vi "ReadForceIni2#.vi"(1 "configuration file path":path=path "E:/LabVIEW/福尔达/AppData") -> ()   [LabVIEW 2018]
uses:
  <vilib>/Utility/config.llb/Read Key (String).vi
  <vilib>/Utility/config.llb/Read Key (Double).vi
  <vilib>/Utility/config.llb/NI_LVConfig.lvlib
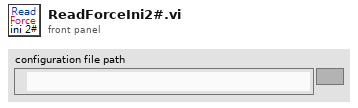
[diagram p1: front panel]
types:
  T1 = typedef "NI_LVConfig.lvlib/Config Data RefNum.ctl" = refnum<k1>
  T2 = cluster{"选择":enum16{"Fx", "Fy", "Fz", "Mx", "My", "Mz"}, "系数x":sgl, "系数+":sgl, "上限":sgl, "下限":sgl, "Ymax":dbl, "Ymin":dbl, "点数":dbl, "锁系数x":sgl, "锁上限":sgl, "锁下限":sgl, "锁系数+":sgl, "起点":dbl, "终点":dbl, "锁起点":dbl, "锁终点":dbl, "上参考":sgl, "下参考":sgl, "基准":sgl}
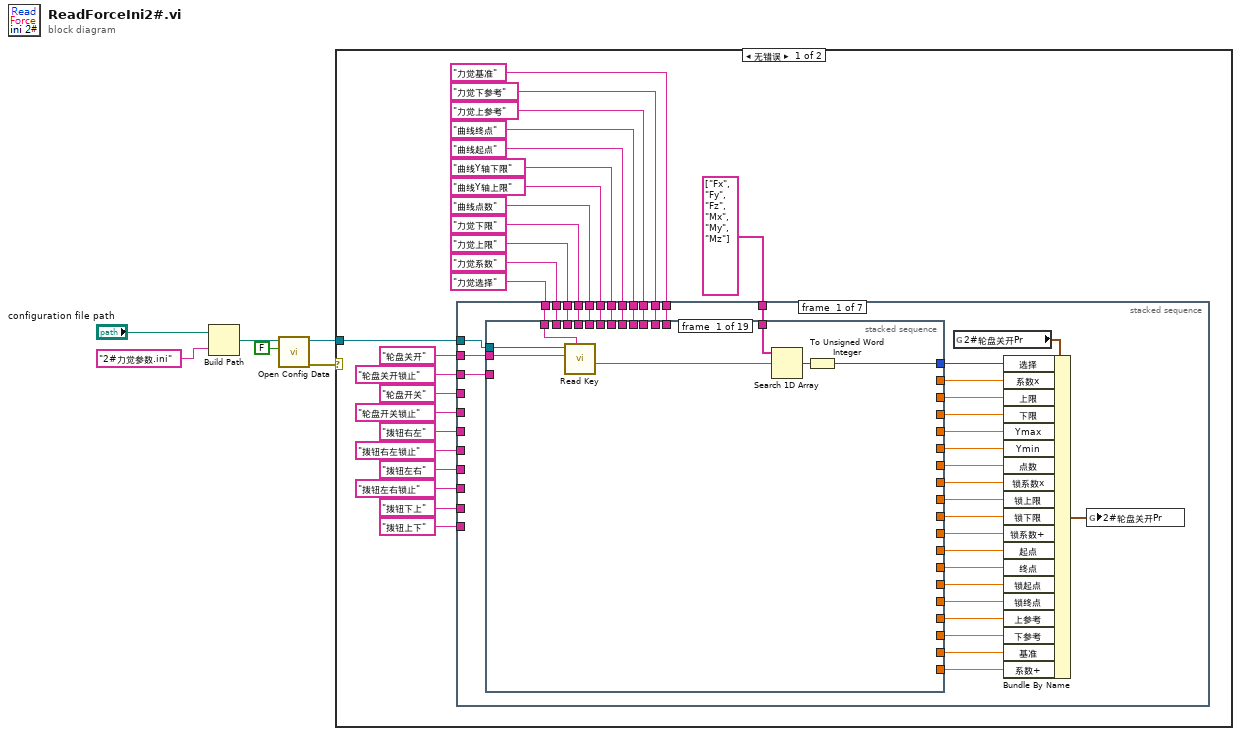
[diagram p0: block diagram]
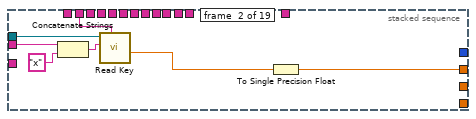
[diagram p2: hidden frame]
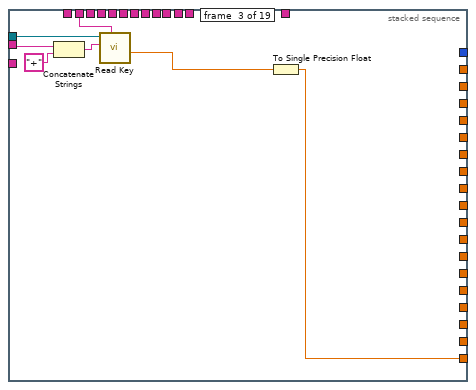
[diagram p3: hidden frame]
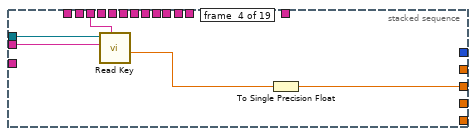
[diagram p4: hidden frame]
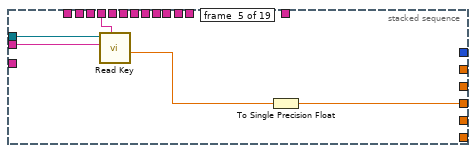
[diagram p5: hidden frame]
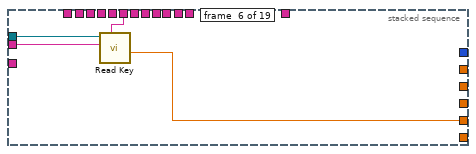
[diagram p6: hidden frame]
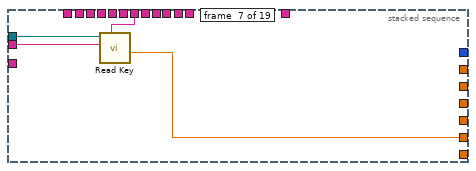
[diagram p7: hidden frame]
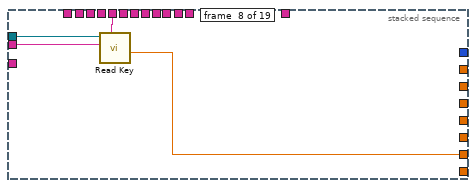
[diagram p8: hidden frame]
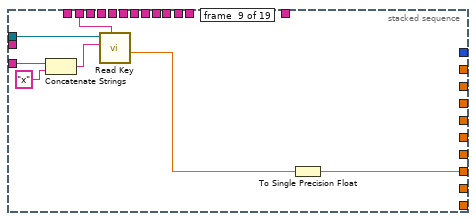
[diagram p9: hidden frame]
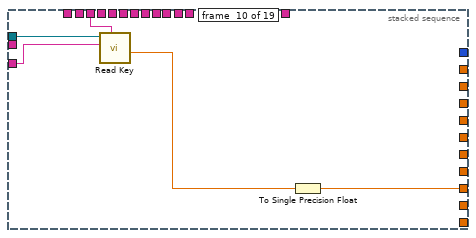
[diagram p10: hidden frame]
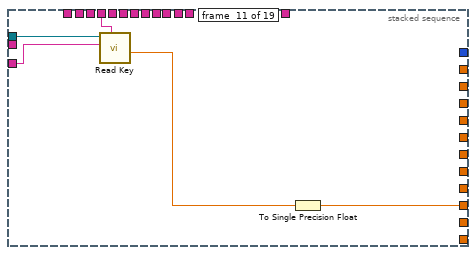
[diagram p11: hidden frame]
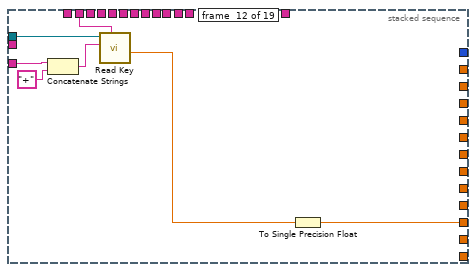
[diagram p12: hidden frame]
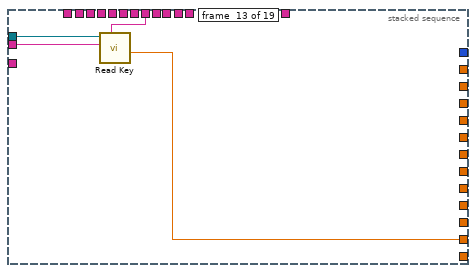
[diagram p13: hidden frame]
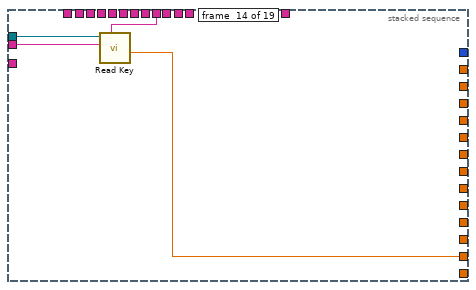
[diagram p14: hidden frame]
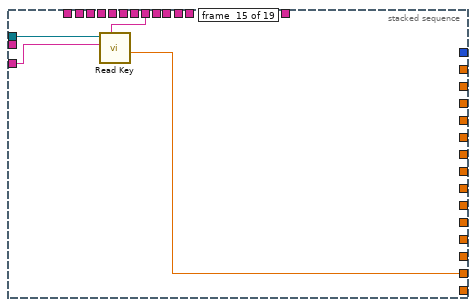
[diagram p15: hidden frame]
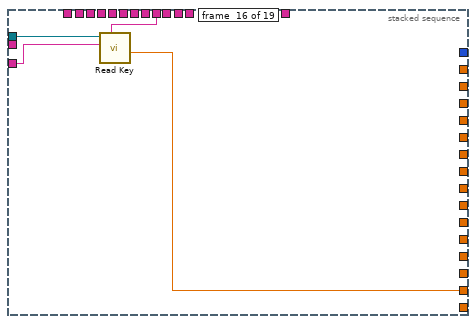
[diagram p16: hidden frame]
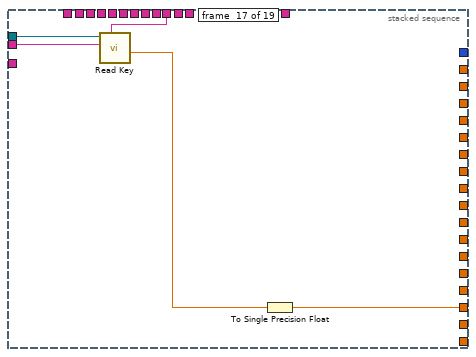
[diagram p17: hidden frame]
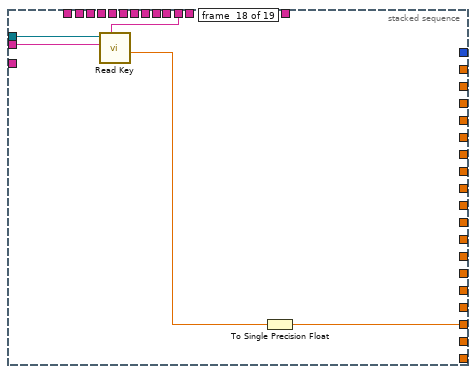
[diagram p18: hidden frame]
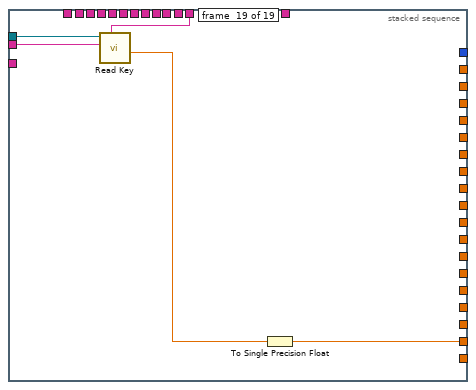
[diagram p19: hidden frame]
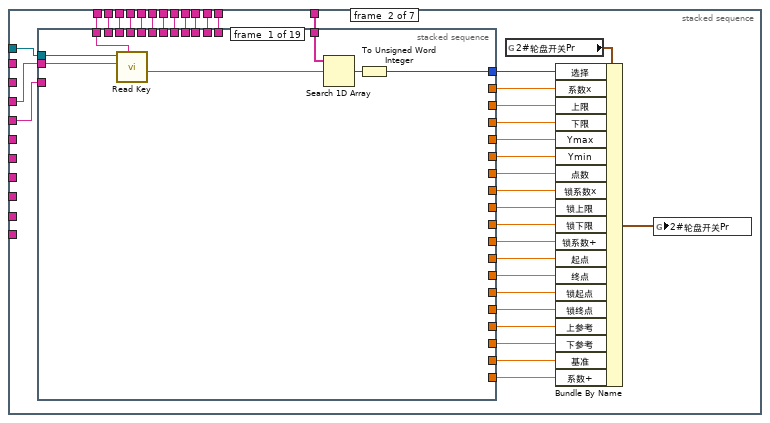
[diagram p20: hidden frame]
diagram:
  n1 = Build Path(base path="configuration file path", name or relative path="2#力觉参数.ini" ("名称或相对路径")) -> (appended path=w3:path)
  n2 = call <vilib>:"Open Config Data.vi"("create file if necessary (T)"=FALSE, "configuration file path"=w3) -> ("error out"=w1:errorcluster, "refnum"=w5:T1)  [unwired: 7 in, 1 out]
  n3 = case shown="无错误" w1 {
    tunnel: w5 -> [w12 w765]
    frame No Error {
      n4 = stacked-sequence {
        tunnel: string[] ["Fx", "Fy", "Fz", "Mx", "My", "Mz"] -> [w67 w202 w337 w472 w600 w696 _]
        tunnel: "轮盘关开" -> [w62 _ _ _ _ _ _]
        tunnel: w12 -> [w66 w201 w336 w471 w599 w695 w763]
        tunnel: "力觉选择" -> [w61 w197 w332 w467 w595 w691 _]
        tunnel: "力觉系数" -> [w60 w196 w331 w466 w594 w690 _]
        tunnel: "力觉上限" -> [w59 w195 w330 w465 w593 w689 _]
        tunnel: "力觉下限" -> [w58 w194 w329 w464 w592 w688 _]
        tunnel: "曲线点数" -> [w57 w193 w328 w463 w591 w687 _]
        tunnel: "曲线Y轴上限" -> [w56 w192 w327 w462 w590 w686 _]
        tunnel: "曲线Y轴下限" -> [w55 w191 w326 w461 w589 w685 _]
        tunnel: "拨钮下上" -> [_ _ _ _ w571 _ _]
        tunnel: "拨钮上下" -> [_ _ _ _ _ w667 _]
        tunnel: "曲线起点" -> [w54 w190 w325 w460 w588 w684 _]
        tunnel: "曲线终点" -> [w53 w189 w324 w459 w587 w683 _]
        tunnel: "力觉上参考" -> [w38 w174 w309 w444 w578 w674 _]
        tunnel: "力觉下参考" -> [w37 w173 w308 w443 w575 w671 _]
        tunnel: "力觉基准" -> [w33 w169 w304 w439 w573 w669 _]
        tunnel: "轮盘关开锁止" -> [w31 _ _ _ _ _ _]
        tunnel: "轮盘开关" -> [_ w167 _ _ _ _ _]
        tunnel: "轮盘开关锁止" -> [_ w166 _ _ _ _ _]
        tunnel: "拨钮右左" -> [_ _ w302 _ _ _ _]
        tunnel: "拨钮左右" -> [_ _ _ w437 _ _ _]
        tunnel: "拨钮左右锁止" -> [_ _ _ w436 _ _ _]
        tunnel: "拨钮右左锁止" -> [_ _ w301 _ _ _ _]
        frame #0 {
          n5 = stacked-sequence {
            tunnel: w67 -> [w74 _ _ _ _ _ _ _ _ _ _ _ _ _ _ _ _ _ _]
            tunnel: w62 -> [w72 w76 w83 w93 w98 w102 w106 w110 _ _ _ _ w135 w139 _ _ w154 w159 w164]
            tunnel: w66 -> [w71 w81 w88 w92 w97 w101 w105 w109 w117 w122 w127 w134 w138 w142 w146 w150 w155 w160 w165]
            tunnel: [w70 _ _ _ _ _ _ _ _ _ _ _ _ _ _ _ _ _ _] -> w64
            tunnel: w61 -> [w68 _ _ _ _ _ _ _ _ _ _ _ _ _ _ _ _ _ _]
            tunnel: w60 -> [_ w80 w87 _ _ _ _ _ w116 _ _ w129 _ _ _ _ _ _ _]
            tunnel: w59 -> [_ _ _ w89 _ _ _ _ _ w119 _ _ _ _ _ _ _ _ _]
            tunnel: w58 -> [_ _ _ _ w94 _ _ _ _ _ w124 _ _ _ _ _ _ _ _]
            tunnel: w57 -> [_ _ _ _ _ _ _ w108 _ _ _ _ _ _ _ _ _ _ _]
            tunnel: w56 -> [_ _ _ _ _ w100 _ _ _ _ _ _ _ _ _ _ _ _ _]
            tunnel: w55 -> [_ _ _ _ _ _ w103 _ _ _ _ _ _ _ _ _ _ _ _]
            tunnel: w54 -> [_ _ _ _ _ _ _ _ _ _ _ _ w137 _ w144 _ _ _ _]
            tunnel: w53 -> [_ _ _ _ _ _ _ _ _ _ _ _ _ w140 _ w149 _ _ _]
            tunnel: [_ w78 _ _ _ _ _ _ _ _ _ _ _ _ _ _ _ _ _] -> w52
            tunnel: [_ _ _ w90 _ _ _ _ _ _ _ _ _ _ _ _ _ _ _] -> w51
            tunnel: [_ _ _ _ w95 _ _ _ _ _ _ _ _ _ _ _ _ _ _] -> w50
            tunnel: [_ _ _ _ _ w99 _ _ _ _ _ _ _ _ _ _ _ _ _] -> w49
            tunnel: [_ _ _ _ _ _ w104 _ _ _ _ _ _ _ _ _ _ _ _] -> w48
            tunnel: [_ _ _ _ _ _ _ w107 _ _ _ _ _ _ _ _ _ _ _] -> w47
            tunnel: [_ _ _ _ _ _ _ _ w113 _ _ _ _ _ _ _ _ _ _] -> w46
            tunnel: [_ _ _ _ _ _ _ _ _ w120 _ _ _ _ _ _ _ _ _] -> w45
            tunnel: [_ _ _ _ _ _ _ _ _ _ w125 _ _ _ _ _ _ _ _] -> w44
            tunnel: [_ _ _ _ _ _ _ _ _ _ _ w132 _ _ _ _ _ _ _] -> w43
            tunnel: [_ _ _ _ _ _ _ _ _ _ _ _ w136 _ _ _ _ _ _] -> w42
            tunnel: [_ _ _ _ _ _ _ _ _ _ _ _ _ w141 _ _ _ _ _] -> w41
            tunnel: [_ _ _ _ _ _ _ _ _ _ _ _ _ _ w145 _ _ _ _] -> w40
            tunnel: [_ _ _ _ _ _ _ _ _ _ _ _ _ _ _ w148 _ _ _] -> w39
            tunnel: w38 -> [_ _ _ _ _ _ _ _ _ _ _ _ _ _ _ _ w151 _ _]
            tunnel: w37 -> [_ _ _ _ _ _ _ _ _ _ _ _ _ _ _ _ _ w157 _]
            tunnel: [_ _ _ _ _ _ _ _ _ _ _ _ _ _ _ _ w153 _ _] -> w36
            tunnel: [_ _ _ _ _ _ _ _ _ _ _ _ _ _ _ _ _ w156 _] -> w35
            tunnel: [_ _ _ _ _ _ _ _ _ _ _ _ _ _ _ _ _ _ w162] -> w34
            tunnel: w33 -> [_ _ _ _ _ _ _ _ _ _ _ _ _ _ _ _ _ _ w161]
            tunnel: [_ _ w85 _ _ _ _ _ _ _ _ _ _ _ _ _ _ _ _] -> w32
            tunnel: w31 -> [_ _ _ _ _ _ _ _ w111 w118 w123 w128 _ _ w143 w147 _ _ _]
            frame #0 {
              n6 = call-poly <vilib>:"Read Key.vi"("section"=w68, "key"=w72, "refnum"=w71) -> ("value"=w73:string)  [unwired: 5 in, 3 out]
              n7 = Search 1D Array(1D array=w74, element=w73) -> (index of element=w69:i32)  [unwired: 1 in]
              n8 = To Unsigned Word Integer(number=w69) -> (unsigned 16bit integer=w70:u16)
            }
            frame #1 {
              n9 = Concatenate Strings(w76, "x") -> (w75:string)
              n10 = call-poly <vilib>:"Read Key.vi"("section"=w80, "key"=w75, "refnum"=w81) -> ("value"=w79:dbl)  [unwired: 5 in, 3 out]
              n11 = To Single Precision Float(number=w79) -> (single precision float=w78:sgl)
            }
            frame #2 {
              n12 = Concatenate Strings(w83, "+") -> (w82:string)
              n13 = call-poly <vilib>:"Read Key.vi"("section"=w87, "key"=w82, "refnum"=w88) -> ("value"=w86:dbl)  [unwired: 5 in, 3 out]
              n14 = To Single Precision Float(number=w86) -> (single precision float=w85:sgl)
            }
            frame #3 {
              n15 = call-poly <vilib>:"Read Key.vi"("section"=w89, "key"=w93, "refnum"=w92) -> ("value"=w91:dbl)  [unwired: 5 in, 3 out]
              n16 = To Single Precision Float(number=w91) -> (single precision float=w90:sgl)
            }
            frame #4 {
              n17 = call-poly <vilib>:"Read Key.vi"("section"=w94, "key"=w98, "refnum"=w97) -> ("value"=w96:dbl)  [unwired: 5 in, 3 out]
              n18 = To Single Precision Float(number=w96) -> (single precision float=w95:sgl)
            }
            frame #5 {
              n19 = call-poly <vilib>:"Read Key.vi"("section"=w100, "key"=w102, "refnum"=w101) -> ("value"=w99:dbl)  [unwired: 5 in, 3 out]
            }
            frame #6 {
              n20 = call-poly <vilib>:"Read Key.vi"("section"=w103, "key"=w106, "refnum"=w105) -> ("value"=w104:dbl)  [unwired: 5 in, 3 out]
            }
            frame #7 {
              n21 = call-poly <vilib>:"Read Key.vi"("section"=w108, "key"=w110, "refnum"=w109) -> ("value"=w107:dbl)  [unwired: 5 in, 3 out]
            }
            frame #8 {
              n22 = Concatenate Strings(w111, "x") -> (w115:string)
              n23 = call-poly <vilib>:"Read Key.vi"("section"=w116, "key"=w115, "refnum"=w117) -> ("value"=w112:dbl)  [unwired: 5 in, 3 out]
              n24 = To Single Precision Float(number=w112) -> (single precision float=w113:sgl)
            }
            frame #9 {
              n25 = call-poly <vilib>:"Read Key.vi"("section"=w119, "key"=w118, "refnum"=w122) -> ("value"=w121:dbl)  [unwired: 5 in, 3 out]
              n26 = To Single Precision Float(number=w121) -> (single precision float=w120:sgl)
            }
            frame #10 {
              n27 = call-poly <vilib>:"Read Key.vi"("section"=w124, "key"=w123, "refnum"=w127) -> ("value"=w126:dbl)  [unwired: 5 in, 3 out]
              n28 = To Single Precision Float(number=w126) -> (single precision float=w125:sgl)
            }
            frame #11 {
              n29 = Concatenate Strings(w128, "+") -> (w131:string)
              n30 = call-poly <vilib>:"Read Key.vi"("section"=w129, "key"=w131, "refnum"=w134) -> ("value"=w133:dbl)  [unwired: 5 in, 3 out]
              n31 = To Single Precision Float(number=w133) -> (single precision float=w132:sgl)
            }
            frame #12 {
              n32 = call-poly <vilib>:"Read Key.vi"("section"=w137, "key"=w135, "refnum"=w138) -> ("value"=w136:dbl)  [unwired: 5 in, 3 out]
            }
            frame #13 {
              n33 = call-poly <vilib>:"Read Key.vi"("section"=w140, "key"=w139, "refnum"=w142) -> ("value"=w141:dbl)  [unwired: 5 in, 3 out]
            }
            frame #14 {
              n34 = call-poly <vilib>:"Read Key.vi"("section"=w144, "key"=w143, "refnum"=w146) -> ("value"=w145:dbl)  [unwired: 5 in, 3 out]
            }
            frame #15 {
              n35 = call-poly <vilib>:"Read Key.vi"("section"=w149, "key"=w147, "refnum"=w150) -> ("value"=w148:dbl)  [unwired: 5 in, 3 out]
            }
            frame #16 {
              n36 = call-poly <vilib>:"Read Key.vi"("section"=w151, "key"=w154, "refnum"=w155) -> ("value"=w152:dbl)  [unwired: 5 in, 3 out]
              n37 = To Single Precision Float(number=w152) -> (single precision float=w153:sgl)
            }
            frame #17 {
              n38 = call-poly <vilib>:"Read Key.vi"("section"=w157, "key"=w159, "refnum"=w160) -> ("value"=w158:dbl)  [unwired: 5 in, 3 out]
              n39 = To Single Precision Float(number=w158) -> (single precision float=w156:sgl)
            }
            frame #18 {
              n40 = call-poly <vilib>:"Read Key.vi"("section"=w161, "key"=w164, "refnum"=w165) -> ("value"=w163:dbl)  [unwired: 5 in, 3 out]
              n41 = To Single Precision Float(number=w163) -> (single precision float=w162:sgl)
            }
          }
          n42 = global read "全局F参数.vi" "2#轮盘关开Pr"() -> (w65:T2)
          n43 = Bundle By Name(cluster=w65, "选择"=w64, "系数x"=w52, "上限"=w51, "下限"=w50, "Ymax"=w49, "Ymin"=w48, "点数"=w47, "锁系数x"=w46, "锁上限"=w45, "锁下限"=w44, "锁系数+"=w43, "起点"=w42, "终点"=w41, "锁起点"=w40, "锁终点"=w39, "上参考"=w36, "下参考"=w35, "基准"=w34, "系数+"=w32) -> (w63:T2)
          n44 = global write "全局F参数.vi" "2#轮盘关开Pr"(w63) -> ()
        }
        frame #1 {
          n45 = stacked-sequence {
            tunnel: w202 -> [w209 _ _ _ _ _ _ _ _ _ _ _ _ _ _ _ _ _ _]
            tunnel: w167 -> [w207 w211 w218 w228 w233 w237 w241 w245 _ _ _ _ w270 w274 _ _ w289 w294 w299]
            tunnel: w201 -> [w206 w216 w223 w227 w232 w236 w240 w244 w252 w257 w262 w269 w273 w277 w281 w285 w290 w295 w300]
            tunnel: [w205 _ _ _ _ _ _ _ _ _ _ _ _ _ _ _ _ _ _] -> w199
            tunnel: w197 -> [w203 _ _ _ _ _ _ _ _ _ _ _ _ _ _ _ _ _ _]
            tunnel: w196 -> [_ w215 w222 _ _ _ _ _ w251 _ _ w264 _ _ _ _ _ _ _]
            tunnel: w195 -> [_ _ _ w224 _ _ _ _ _ w254 _ _ _ _ _ _ _ _ _]
            tunnel: w194 -> [_ _ _ _ w229 _ _ _ _ _ w259 _ _ _ _ _ _ _ _]
            tunnel: w193 -> [_ _ _ _ _ _ _ w243 _ _ _ _ _ _ _ _ _ _ _]
            tunnel: w192 -> [_ _ _ _ _ w235 _ _ _ _ _ _ _ _ _ _ _ _ _]
            tunnel: w191 -> [_ _ _ _ _ _ w238 _ _ _ _ _ _ _ _ _ _ _ _]
            tunnel: w190 -> [_ _ _ _ _ _ _ _ _ _ _ _ w272 _ w279 _ _ _ _]
            tunnel: w189 -> [_ _ _ _ _ _ _ _ _ _ _ _ _ w275 _ w284 _ _ _]
            tunnel: [_ w213 _ _ _ _ _ _ _ _ _ _ _ _ _ _ _ _ _] -> w188
            tunnel: [_ _ _ w225 _ _ _ _ _ _ _ _ _ _ _ _ _ _ _] -> w187
            tunnel: [_ _ _ _ w230 _ _ _ _ _ _ _ _ _ _ _ _ _ _] -> w186
            tunnel: [_ _ _ _ _ w234 _ _ _ _ _ _ _ _ _ _ _ _ _] -> w185
            tunnel: [_ _ _ _ _ _ w239 _ _ _ _ _ _ _ _ _ _ _ _] -> w184
            tunnel: [_ _ _ _ _ _ _ w242 _ _ _ _ _ _ _ _ _ _ _] -> w183
            tunnel: [_ _ _ _ _ _ _ _ w248 _ _ _ _ _ _ _ _ _ _] -> w182
            tunnel: [_ _ _ _ _ _ _ _ _ w255 _ _ _ _ _ _ _ _ _] -> w181
            tunnel: [_ _ _ _ _ _ _ _ _ _ w260 _ _ _ _ _ _ _ _] -> w180
            tunnel: [_ _ _ _ _ _ _ _ _ _ _ w267 _ _ _ _ _ _ _] -> w179
            tunnel: [_ _ _ _ _ _ _ _ _ _ _ _ w271 _ _ _ _ _ _] -> w178
            tunnel: [_ _ _ _ _ _ _ _ _ _ _ _ _ w276 _ _ _ _ _] -> w177
            tunnel: [_ _ _ _ _ _ _ _ _ _ _ _ _ _ w280 _ _ _ _] -> w176
            tunnel: [_ _ _ _ _ _ _ _ _ _ _ _ _ _ _ w283 _ _ _] -> w175
            tunnel: w174 -> [_ _ _ _ _ _ _ _ _ _ _ _ _ _ _ _ w286 _ _]
            tunnel: w173 -> [_ _ _ _ _ _ _ _ _ _ _ _ _ _ _ _ _ w292 _]
            tunnel: [_ _ _ _ _ _ _ _ _ _ _ _ _ _ _ _ w288 _ _] -> w172
            tunnel: [_ _ _ _ _ _ _ _ _ _ _ _ _ _ _ _ _ w291 _] -> w171
            tunnel: [_ _ _ _ _ _ _ _ _ _ _ _ _ _ _ _ _ _ w297] -> w170
            tunnel: w169 -> [_ _ _ _ _ _ _ _ _ _ _ _ _ _ _ _ _ _ w296]
            tunnel: [_ _ w220 _ _ _ _ _ _ _ _ _ _ _ _ _ _ _ _] -> w168
            tunnel: w166 -> [_ _ _ _ _ _ _ _ w246 w253 w258 w263 _ _ w278 w282 _ _ _]
            frame #0 {
              n46 = call-poly <vilib>:"Read Key.vi"("section"=w203, "key"=w207, "refnum"=w206) -> ("value"=w208:string)  [unwired: 5 in, 3 out]
              n47 = Search 1D Array(1D array=w209, element=w208) -> (index of element=w204:i32)  [unwired: 1 in]
              n48 = To Unsigned Word Integer(number=w204) -> (unsigned 16bit integer=w205:u16)
            }
            frame #1 {
              n49 = Concatenate Strings(w211, "x") -> (w210:string)
              n50 = call-poly <vilib>:"Read Key.vi"("section"=w215, "key"=w210, "refnum"=w216) -> ("value"=w214:dbl)  [unwired: 5 in, 3 out]
              n51 = To Single Precision Float(number=w214) -> (single precision float=w213:sgl)
            }
            frame #2 {
              n52 = Concatenate Strings(w218, "+") -> (w217:string)
              n53 = call-poly <vilib>:"Read Key.vi"("section"=w222, "key"=w217, "refnum"=w223) -> ("value"=w221:dbl)  [unwired: 5 in, 3 out]
              n54 = To Single Precision Float(number=w221) -> (single precision float=w220:sgl)
            }
            frame #3 {
              n55 = call-poly <vilib>:"Read Key.vi"("section"=w224, "key"=w228, "refnum"=w227) -> ("value"=w226:dbl)  [unwired: 5 in, 3 out]
              n56 = To Single Precision Float(number=w226) -> (single precision float=w225:sgl)
            }
            frame #4 {
              n57 = call-poly <vilib>:"Read Key.vi"("section"=w229, "key"=w233, "refnum"=w232) -> ("value"=w231:dbl)  [unwired: 5 in, 3 out]
              n58 = To Single Precision Float(number=w231) -> (single precision float=w230:sgl)
            }
            frame #5 {
              n59 = call-poly <vilib>:"Read Key.vi"("section"=w235, "key"=w237, "refnum"=w236) -> ("value"=w234:dbl)  [unwired: 5 in, 3 out]
            }
            frame #6 {
              n60 = call-poly <vilib>:"Read Key.vi"("section"=w238, "key"=w241, "refnum"=w240) -> ("value"=w239:dbl)  [unwired: 5 in, 3 out]
            }
            frame #7 {
              n61 = call-poly <vilib>:"Read Key.vi"("section"=w243, "key"=w245, "refnum"=w244) -> ("value"=w242:dbl)  [unwired: 5 in, 3 out]
            }
            frame #8 {
              n62 = Concatenate Strings(w246, "x") -> (w250:string)
              n63 = call-poly <vilib>:"Read Key.vi"("section"=w251, "key"=w250, "refnum"=w252) -> ("value"=w247:dbl)  [unwired: 5 in, 3 out]
              n64 = To Single Precision Float(number=w247) -> (single precision float=w248:sgl)
            }
            frame #9 {
              n65 = call-poly <vilib>:"Read Key.vi"("section"=w254, "key"=w253, "refnum"=w257) -> ("value"=w256:dbl)  [unwired: 5 in, 3 out]
              n66 = To Single Precision Float(number=w256) -> (single precision float=w255:sgl)
            }
            frame #10 {
              n67 = call-poly <vilib>:"Read Key.vi"("section"=w259, "key"=w258, "refnum"=w262) -> ("value"=w261:dbl)  [unwired: 5 in, 3 out]
              n68 = To Single Precision Float(number=w261) -> (single precision float=w260:sgl)
            }
            frame #11 {
              n69 = Concatenate Strings(w263, "+") -> (w266:string)
              n70 = call-poly <vilib>:"Read Key.vi"("section"=w264, "key"=w266, "refnum"=w269) -> ("value"=w268:dbl)  [unwired: 5 in, 3 out]
              n71 = To Single Precision Float(number=w268) -> (single precision float=w267:sgl)
            }
            frame #12 {
              n72 = call-poly <vilib>:"Read Key.vi"("section"=w272, "key"=w270, "refnum"=w273) -> ("value"=w271:dbl)  [unwired: 5 in, 3 out]
            }
            frame #13 {
              n73 = call-poly <vilib>:"Read Key.vi"("section"=w275, "key"=w274, "refnum"=w277) -> ("value"=w276:dbl)  [unwired: 5 in, 3 out]
            }
            frame #14 {
              n74 = call-poly <vilib>:"Read Key.vi"("section"=w279, "key"=w278, "refnum"=w281) -> ("value"=w280:dbl)  [unwired: 5 in, 3 out]
            }
            frame #15 {
              n75 = call-poly <vilib>:"Read Key.vi"("section"=w284, "key"=w282, "refnum"=w285) -> ("value"=w283:dbl)  [unwired: 5 in, 3 out]
            }
            frame #16 {
              n76 = call-poly <vilib>:"Read Key.vi"("section"=w286, "key"=w289, "refnum"=w290) -> ("value"=w287:dbl)  [unwired: 5 in, 3 out]
              n77 = To Single Precision Float(number=w287) -> (single precision float=w288:sgl)
            }
            frame #17 {
              n78 = call-poly <vilib>:"Read Key.vi"("section"=w292, "key"=w294, "refnum"=w295) -> ("value"=w293:dbl)  [unwired: 5 in, 3 out]
              n79 = To Single Precision Float(number=w293) -> (single precision float=w291:sgl)
            }
            frame #18 {
              n80 = call-poly <vilib>:"Read Key.vi"("section"=w296, "key"=w299, "refnum"=w300) -> ("value"=w298:dbl)  [unwired: 5 in, 3 out]
              n81 = To Single Precision Float(number=w298) -> (single precision float=w297:sgl)
            }
          }
          n82 = global read "全局F参数.vi" "2#轮盘开关Pr"() -> (w200:T2)
          n83 = Bundle By Name(cluster=w200, "选择"=w199, "系数x"=w188, "上限"=w187, "下限"=w186, "Ymax"=w185, "Ymin"=w184, "点数"=w183, "锁系数x"=w182, "锁上限"=w181, "锁下限"=w180, "锁系数+"=w179, "起点"=w178, "终点"=w177, "锁起点"=w176, "锁终点"=w175, "上参考"=w172, "下参考"=w171, "基准"=w170, "系数+"=w168) -> (w198:T2)
          n84 = global write "全局F参数.vi" "2#轮盘开关Pr"(w198) -> ()
        }
        frame #2 {
          n85 = stacked-sequence {
            tunnel: w337 -> [w344 _ _ _ _ _ _ _ _ _ _ _ _ _ _ _ _ _ _]
            tunnel: w302 -> [w342 w346 w353 w363 w368 w372 w376 w380 _ _ _ _ w405 w409 _ _ w424 w429 w434]
            tunnel: w336 -> [w341 w351 w358 w362 w367 w371 w375 w379 w387 w392 w397 w404 w408 w412 w416 w420 w425 w430 w435]
            tunnel: [w340 _ _ _ _ _ _ _ _ _ _ _ _ _ _ _ _ _ _] -> w334
            tunnel: w332 -> [w338 _ _ _ _ _ _ _ _ _ _ _ _ _ _ _ _ _ _]
            tunnel: w331 -> [_ w350 w357 _ _ _ _ _ w386 _ _ w399 _ _ _ _ _ _ _]
            tunnel: w330 -> [_ _ _ w359 _ _ _ _ _ w389 _ _ _ _ _ _ _ _ _]
            tunnel: w329 -> [_ _ _ _ w364 _ _ _ _ _ w394 _ _ _ _ _ _ _ _]
            tunnel: w328 -> [_ _ _ _ _ _ _ w378 _ _ _ _ _ _ _ _ _ _ _]
            tunnel: w327 -> [_ _ _ _ _ w370 _ _ _ _ _ _ _ _ _ _ _ _ _]
            tunnel: w326 -> [_ _ _ _ _ _ w373 _ _ _ _ _ _ _ _ _ _ _ _]
            tunnel: w325 -> [_ _ _ _ _ _ _ _ _ _ _ _ w407 _ w414 _ _ _ _]
            tunnel: w324 -> [_ _ _ _ _ _ _ _ _ _ _ _ _ w410 _ w419 _ _ _]
            tunnel: [_ w348 _ _ _ _ _ _ _ _ _ _ _ _ _ _ _ _ _] -> w323
            tunnel: [_ _ _ w360 _ _ _ _ _ _ _ _ _ _ _ _ _ _ _] -> w322
            tunnel: [_ _ _ _ w365 _ _ _ _ _ _ _ _ _ _ _ _ _ _] -> w321
            tunnel: [_ _ _ _ _ w369 _ _ _ _ _ _ _ _ _ _ _ _ _] -> w320
            tunnel: [_ _ _ _ _ _ w374 _ _ _ _ _ _ _ _ _ _ _ _] -> w319
            tunnel: [_ _ _ _ _ _ _ w377 _ _ _ _ _ _ _ _ _ _ _] -> w318
            tunnel: [_ _ _ _ _ _ _ _ w383 _ _ _ _ _ _ _ _ _ _] -> w317
            tunnel: [_ _ _ _ _ _ _ _ _ w390 _ _ _ _ _ _ _ _ _] -> w316
            tunnel: [_ _ _ _ _ _ _ _ _ _ w395 _ _ _ _ _ _ _ _] -> w315
            tunnel: [_ _ _ _ _ _ _ _ _ _ _ w402 _ _ _ _ _ _ _] -> w314
            tunnel: [_ _ _ _ _ _ _ _ _ _ _ _ w406 _ _ _ _ _ _] -> w313
            tunnel: [_ _ _ _ _ _ _ _ _ _ _ _ _ w411 _ _ _ _ _] -> w312
            tunnel: [_ _ _ _ _ _ _ _ _ _ _ _ _ _ w415 _ _ _ _] -> w311
            tunnel: [_ _ _ _ _ _ _ _ _ _ _ _ _ _ _ w418 _ _ _] -> w310
            tunnel: w309 -> [_ _ _ _ _ _ _ _ _ _ _ _ _ _ _ _ w421 _ _]
            tunnel: w308 -> [_ _ _ _ _ _ _ _ _ _ _ _ _ _ _ _ _ w427 _]
            tunnel: [_ _ _ _ _ _ _ _ _ _ _ _ _ _ _ _ w423 _ _] -> w307
            tunnel: [_ _ _ _ _ _ _ _ _ _ _ _ _ _ _ _ _ w426 _] -> w306
            tunnel: [_ _ _ _ _ _ _ _ _ _ _ _ _ _ _ _ _ _ w432] -> w305
            tunnel: w304 -> [_ _ _ _ _ _ _ _ _ _ _ _ _ _ _ _ _ _ w431]
            tunnel: [_ _ w355 _ _ _ _ _ _ _ _ _ _ _ _ _ _ _ _] -> w303
            tunnel: w301 -> [_ _ _ _ _ _ _ _ w381 w388 w393 w398 _ _ w413 w417 _ _ _]
            frame #0 {
              n86 = call-poly <vilib>:"Read Key.vi"("section"=w338, "key"=w342, "refnum"=w341) -> ("value"=w343:string)  [unwired: 5 in, 3 out]
              n87 = Search 1D Array(1D array=w344, element=w343) -> (index of element=w339:i32)  [unwired: 1 in]
              n88 = To Unsigned Word Integer(number=w339) -> (unsigned 16bit integer=w340:u16)
            }
            frame #1 {
              n89 = Concatenate Strings(w346, "x") -> (w345:string)
              n90 = call-poly <vilib>:"Read Key.vi"("section"=w350, "key"=w345, "refnum"=w351) -> ("value"=w349:dbl)  [unwired: 5 in, 3 out]
              n91 = To Single Precision Float(number=w349) -> (single precision float=w348:sgl)
            }
            frame #2 {
              n92 = Concatenate Strings(w353, "+") -> (w352:string)
              n93 = call-poly <vilib>:"Read Key.vi"("section"=w357, "key"=w352, "refnum"=w358) -> ("value"=w356:dbl)  [unwired: 5 in, 3 out]
              n94 = To Single Precision Float(number=w356) -> (single precision float=w355:sgl)
            }
            frame #3 {
              n95 = call-poly <vilib>:"Read Key.vi"("section"=w359, "key"=w363, "refnum"=w362) -> ("value"=w361:dbl)  [unwired: 5 in, 3 out]
              n96 = To Single Precision Float(number=w361) -> (single precision float=w360:sgl)
            }
            frame #4 {
              n97 = call-poly <vilib>:"Read Key.vi"("section"=w364, "key"=w368, "refnum"=w367) -> ("value"=w366:dbl)  [unwired: 5 in, 3 out]
              n98 = To Single Precision Float(number=w366) -> (single precision float=w365:sgl)
            }
            frame #5 {
              n99 = call-poly <vilib>:"Read Key.vi"("section"=w370, "key"=w372, "refnum"=w371) -> ("value"=w369:dbl)  [unwired: 5 in, 3 out]
            }
            frame #6 {
              n100 = call-poly <vilib>:"Read Key.vi"("section"=w373, "key"=w376, "refnum"=w375) -> ("value"=w374:dbl)  [unwired: 5 in, 3 out]
            }
            frame #7 {
              n101 = call-poly <vilib>:"Read Key.vi"("section"=w378, "key"=w380, "refnum"=w379) -> ("value"=w377:dbl)  [unwired: 5 in, 3 out]
            }
            frame #8 {
              n102 = Concatenate Strings(w381, "x") -> (w385:string)
              n103 = call-poly <vilib>:"Read Key.vi"("section"=w386, "key"=w385, "refnum"=w387) -> ("value"=w382:dbl)  [unwired: 5 in, 3 out]
              n104 = To Single Precision Float(number=w382) -> (single precision float=w383:sgl)
            }
            frame #9 {
              n105 = call-poly <vilib>:"Read Key.vi"("section"=w389, "key"=w388, "refnum"=w392) -> ("value"=w391:dbl)  [unwired: 5 in, 3 out]
              n106 = To Single Precision Float(number=w391) -> (single precision float=w390:sgl)
            }
            frame #10 {
              n107 = call-poly <vilib>:"Read Key.vi"("section"=w394, "key"=w393, "refnum"=w397) -> ("value"=w396:dbl)  [unwired: 5 in, 3 out]
              n108 = To Single Precision Float(number=w396) -> (single precision float=w395:sgl)
            }
            frame #11 {
              n109 = Concatenate Strings(w398, "+") -> (w401:string)
              n110 = call-poly <vilib>:"Read Key.vi"("section"=w399, "key"=w401, "refnum"=w404) -> ("value"=w403:dbl)  [unwired: 5 in, 3 out]
              n111 = To Single Precision Float(number=w403) -> (single precision float=w402:sgl)
            }
            frame #12 {
              n112 = call-poly <vilib>:"Read Key.vi"("section"=w407, "key"=w405, "refnum"=w408) -> ("value"=w406:dbl)  [unwired: 5 in, 3 out]
            }
            frame #13 {
              n113 = call-poly <vilib>:"Read Key.vi"("section"=w410, "key"=w409, "refnum"=w412) -> ("value"=w411:dbl)  [unwired: 5 in, 3 out]
            }
            frame #14 {
              n114 = call-poly <vilib>:"Read Key.vi"("section"=w414, "key"=w413, "refnum"=w416) -> ("value"=w415:dbl)  [unwired: 5 in, 3 out]
            }
            frame #15 {
              n115 = call-poly <vilib>:"Read Key.vi"("section"=w419, "key"=w417, "refnum"=w420) -> ("value"=w418:dbl)  [unwired: 5 in, 3 out]
            }
            frame #16 {
              n116 = call-poly <vilib>:"Read Key.vi"("section"=w421, "key"=w424, "refnum"=w425) -> ("value"=w422:dbl)  [unwired: 5 in, 3 out]
              n117 = To Single Precision Float(number=w422) -> (single precision float=w423:sgl)
            }
            frame #17 {
              n118 = call-poly <vilib>:"Read Key.vi"("section"=w427, "key"=w429, "refnum"=w430) -> ("value"=w428:dbl)  [unwired: 5 in, 3 out]
              n119 = To Single Precision Float(number=w428) -> (single precision float=w426:sgl)
            }
            frame #18 {
              n120 = call-poly <vilib>:"Read Key.vi"("section"=w431, "key"=w434, "refnum"=w435) -> ("value"=w433:dbl)  [unwired: 5 in, 3 out]
              n121 = To Single Precision Float(number=w433) -> (single precision float=w432:sgl)
            }
          }
          n122 = global read "全局F参数.vi" "2#拨钮右左Pr"() -> (w335:T2)
          n123 = Bundle By Name(cluster=w335, "选择"=w334, "系数x"=w323, "上限"=w322, "下限"=w321, "Ymax"=w320, "Ymin"=w319, "点数"=w318, "锁系数x"=w317, "锁上限"=w316, "锁下限"=w315, "锁系数+"=w314, "起点"=w313, "终点"=w312, "锁起点"=w311, "锁终点"=w310, "上参考"=w307, "下参考"=w306, "基准"=w305, "系数+"=w303) -> (w333:T2)
          n124 = global write "全局F参数.vi" "2#拨钮右左Pr"(w333) -> ()
        }
        frame #3 {
          n125 = stacked-sequence {
            tunnel: w472 -> [w479 _ _ _ _ _ _ _ _ _ _ _ _ _ _ _ _ _ _]
            tunnel: w437 -> [w477 w481 w488 w498 w503 w507 w511 w515 _ _ _ _ w540 w544 _ _ w559 w564 w569]
            tunnel: w471 -> [w476 w486 w493 w497 w502 w506 w510 w514 w522 w527 w532 w539 w543 w547 w551 w555 w560 w565 w570]
            tunnel: [w475 _ _ _ _ _ _ _ _ _ _ _ _ _ _ _ _ _ _] -> w469
            tunnel: w467 -> [w473 _ _ _ _ _ _ _ _ _ _ _ _ _ _ _ _ _ _]
            tunnel: w466 -> [_ w485 w492 _ _ _ _ _ w521 _ _ w534 _ _ _ _ _ _ _]
            tunnel: w465 -> [_ _ _ w494 _ _ _ _ _ w524 _ _ _ _ _ _ _ _ _]
            tunnel: w464 -> [_ _ _ _ w499 _ _ _ _ _ w529 _ _ _ _ _ _ _ _]
            tunnel: w463 -> [_ _ _ _ _ _ _ w513 _ _ _ _ _ _ _ _ _ _ _]
            tunnel: w462 -> [_ _ _ _ _ w505 _ _ _ _ _ _ _ _ _ _ _ _ _]
            tunnel: w461 -> [_ _ _ _ _ _ w508 _ _ _ _ _ _ _ _ _ _ _ _]
            tunnel: w460 -> [_ _ _ _ _ _ _ _ _ _ _ _ w542 _ w549 _ _ _ _]
            tunnel: w459 -> [_ _ _ _ _ _ _ _ _ _ _ _ _ w545 _ w554 _ _ _]
            tunnel: [_ w483 _ _ _ _ _ _ _ _ _ _ _ _ _ _ _ _ _] -> w458
            tunnel: [_ _ _ w495 _ _ _ _ _ _ _ _ _ _ _ _ _ _ _] -> w457
            tunnel: [_ _ _ _ w500 _ _ _ _ _ _ _ _ _ _ _ _ _ _] -> w456
            tunnel: [_ _ _ _ _ w504 _ _ _ _ _ _ _ _ _ _ _ _ _] -> w455
            tunnel: [_ _ _ _ _ _ w509 _ _ _ _ _ _ _ _ _ _ _ _] -> w454
            tunnel: [_ _ _ _ _ _ _ w512 _ _ _ _ _ _ _ _ _ _ _] -> w453
            tunnel: [_ _ _ _ _ _ _ _ w518 _ _ _ _ _ _ _ _ _ _] -> w452
            tunnel: [_ _ _ _ _ _ _ _ _ w525 _ _ _ _ _ _ _ _ _] -> w451
            tunnel: [_ _ _ _ _ _ _ _ _ _ w530 _ _ _ _ _ _ _ _] -> w450
            tunnel: [_ _ _ _ _ _ _ _ _ _ _ w537 _ _ _ _ _ _ _] -> w449
            tunnel: [_ _ _ _ _ _ _ _ _ _ _ _ w541 _ _ _ _ _ _] -> w448
            tunnel: [_ _ _ _ _ _ _ _ _ _ _ _ _ w546 _ _ _ _ _] -> w447
            tunnel: [_ _ _ _ _ _ _ _ _ _ _ _ _ _ w550 _ _ _ _] -> w446
            tunnel: [_ _ _ _ _ _ _ _ _ _ _ _ _ _ _ w553 _ _ _] -> w445
            tunnel: w444 -> [_ _ _ _ _ _ _ _ _ _ _ _ _ _ _ _ w556 _ _]
            tunnel: w443 -> [_ _ _ _ _ _ _ _ _ _ _ _ _ _ _ _ _ w562 _]
            tunnel: [_ _ _ _ _ _ _ _ _ _ _ _ _ _ _ _ w558 _ _] -> w442
            tunnel: [_ _ _ _ _ _ _ _ _ _ _ _ _ _ _ _ _ w561 _] -> w441
            tunnel: [_ _ _ _ _ _ _ _ _ _ _ _ _ _ _ _ _ _ w567] -> w440
            tunnel: w439 -> [_ _ _ _ _ _ _ _ _ _ _ _ _ _ _ _ _ _ w566]
            tunnel: [_ _ w490 _ _ _ _ _ _ _ _ _ _ _ _ _ _ _ _] -> w438
            tunnel: w436 -> [_ _ _ _ _ _ _ _ w516 w523 w528 w533 _ _ w548 w552 _ _ _]
            frame #0 {
              n126 = call-poly <vilib>:"Read Key.vi"("section"=w473, "key"=w477, "refnum"=w476) -> ("value"=w478:string)  [unwired: 5 in, 3 out]
              n127 = Search 1D Array(1D array=w479, element=w478) -> (index of element=w474:i32)  [unwired: 1 in]
              n128 = To Unsigned Word Integer(number=w474) -> (unsigned 16bit integer=w475:u16)
            }
            frame #1 {
              n129 = Concatenate Strings(w481, "x") -> (w480:string)
              n130 = call-poly <vilib>:"Read Key.vi"("section"=w485, "key"=w480, "refnum"=w486) -> ("value"=w484:dbl)  [unwired: 5 in, 3 out]
              n131 = To Single Precision Float(number=w484) -> (single precision float=w483:sgl)
            }
            frame #2 {
              n132 = Concatenate Strings(w488, "+") -> (w487:string)
              n133 = call-poly <vilib>:"Read Key.vi"("section"=w492, "key"=w487, "refnum"=w493) -> ("value"=w491:dbl)  [unwired: 5 in, 3 out]
              n134 = To Single Precision Float(number=w491) -> (single precision float=w490:sgl)
            }
            frame #3 {
              n135 = call-poly <vilib>:"Read Key.vi"("section"=w494, "key"=w498, "refnum"=w497) -> ("value"=w496:dbl)  [unwired: 5 in, 3 out]
              n136 = To Single Precision Float(number=w496) -> (single precision float=w495:sgl)
            }
            frame #4 {
              n137 = call-poly <vilib>:"Read Key.vi"("section"=w499, "key"=w503, "refnum"=w502) -> ("value"=w501:dbl)  [unwired: 5 in, 3 out]
              n138 = To Single Precision Float(number=w501) -> (single precision float=w500:sgl)
            }
            frame #5 {
              n139 = call-poly <vilib>:"Read Key.vi"("section"=w505, "key"=w507, "refnum"=w506) -> ("value"=w504:dbl)  [unwired: 5 in, 3 out]
            }
            frame #6 {
              n140 = call-poly <vilib>:"Read Key.vi"("section"=w508, "key"=w511, "refnum"=w510) -> ("value"=w509:dbl)  [unwired: 5 in, 3 out]
            }
            frame #7 {
              n141 = call-poly <vilib>:"Read Key.vi"("section"=w513, "key"=w515, "refnum"=w514) -> ("value"=w512:dbl)  [unwired: 5 in, 3 out]
            }
            frame #8 {
              n142 = Concatenate Strings(w516, "x") -> (w520:string)
              n143 = call-poly <vilib>:"Read Key.vi"("section"=w521, "key"=w520, "refnum"=w522) -> ("value"=w517:dbl)  [unwired: 5 in, 3 out]
              n144 = To Single Precision Float(number=w517) -> (single precision float=w518:sgl)
            }
            frame #9 {
              n145 = call-poly <vilib>:"Read Key.vi"("section"=w524, "key"=w523, "refnum"=w527) -> ("value"=w526:dbl)  [unwired: 5 in, 3 out]
              n146 = To Single Precision Float(number=w526) -> (single precision float=w525:sgl)
            }
            frame #10 {
              n147 = call-poly <vilib>:"Read Key.vi"("section"=w529, "key"=w528, "refnum"=w532) -> ("value"=w531:dbl)  [unwired: 5 in, 3 out]
              n148 = To Single Precision Float(number=w531) -> (single precision float=w530:sgl)
            }
            frame #11 {
              n149 = Concatenate Strings(w533, "+") -> (w536:string)
              n150 = call-poly <vilib>:"Read Key.vi"("section"=w534, "key"=w536, "refnum"=w539) -> ("value"=w538:dbl)  [unwired: 5 in, 3 out]
              n151 = To Single Precision Float(number=w538) -> (single precision float=w537:sgl)
            }
            frame #12 {
              n152 = call-poly <vilib>:"Read Key.vi"("section"=w542, "key"=w540, "refnum"=w543) -> ("value"=w541:dbl)  [unwired: 5 in, 3 out]
            }
            frame #13 {
              n153 = call-poly <vilib>:"Read Key.vi"("section"=w545, "key"=w544, "refnum"=w547) -> ("value"=w546:dbl)  [unwired: 5 in, 3 out]
            }
            frame #14 {
              n154 = call-poly <vilib>:"Read Key.vi"("section"=w549, "key"=w548, "refnum"=w551) -> ("value"=w550:dbl)  [unwired: 5 in, 3 out]
            }
            frame #15 {
              n155 = call-poly <vilib>:"Read Key.vi"("section"=w554, "key"=w552, "refnum"=w555) -> ("value"=w553:dbl)  [unwired: 5 in, 3 out]
            }
            frame #16 {
              n156 = call-poly <vilib>:"Read Key.vi"("section"=w556, "key"=w559, "refnum"=w560) -> ("value"=w557:dbl)  [unwired: 5 in, 3 out]
              n157 = To Single Precision Float(number=w557) -> (single precision float=w558:sgl)
            }
            frame #17 {
              n158 = call-poly <vilib>:"Read Key.vi"("section"=w562, "key"=w564, "refnum"=w565) -> ("value"=w563:dbl)  [unwired: 5 in, 3 out]
              n159 = To Single Precision Float(number=w563) -> (single precision float=w561:sgl)
            }
            frame #18 {
              n160 = call-poly <vilib>:"Read Key.vi"("section"=w566, "key"=w569, "refnum"=w570) -> ("value"=w568:dbl)  [unwired: 5 in, 3 out]
              n161 = To Single Precision Float(number=w568) -> (single precision float=w567:sgl)
            }
          }
          n162 = global read "全局F参数.vi" "2#拨钮左右Pr"() -> (w470:T2)
          n163 = Bundle By Name(cluster=w470, "选择"=w469, "系数x"=w458, "上限"=w457, "下限"=w456, "Ymax"=w455, "Ymin"=w454, "点数"=w453, "锁系数x"=w452, "锁上限"=w451, "锁下限"=w450, "锁系数+"=w449, "起点"=w448, "终点"=w447, "锁起点"=w446, "锁终点"=w445, "上参考"=w442, "下参考"=w441, "基准"=w440, "系数+"=w438) -> (w468:T2)
          n164 = global write "全局F参数.vi" "2#拨钮左右Pr"(w468) -> ()
        }
        frame #4 {
          n165 = stacked-sequence {
            tunnel: w600 -> [w607 _ _ _ _ _ _ _ _ _ _ _ _]
            tunnel: w599 -> [w605 w614 w621 w626 w631 w635 w639 w643 w647 w651 w656 w661 w666]
            tunnel: [w604 _ _ _ _ _ _ _ _ _ _ _ _] -> w597
            tunnel: w595 -> [w602 _ _ _ _ _ _ _ _ _ _ _ _]
            tunnel: w594 -> [_ w613 w620 _ _ _ _ _ _ _ _ _ _]
            tunnel: w593 -> [_ _ _ w624 _ _ _ _ _ _ _ _ _]
            tunnel: w592 -> [_ _ _ _ w629 _ _ _ _ _ _ _ _]
            tunnel: w591 -> [_ _ _ _ _ _ _ w642 _ _ _ _ _]
            tunnel: w590 -> [_ _ _ _ _ w634 _ _ _ _ _ _ _]
            tunnel: w589 -> [_ _ _ _ _ _ w638 _ _ _ _ _ _]
            tunnel: w588 -> [_ _ _ _ _ _ _ _ w646 _ _ _ _]
            tunnel: w587 -> [_ _ _ _ _ _ _ _ _ w650 _ _ _]
            tunnel: [_ w611 _ _ _ _ _ _ _ _ _ _ _] -> w586
            tunnel: [_ _ _ w623 _ _ _ _ _ _ _ _ _] -> w585
            tunnel: [_ _ _ _ w628 _ _ _ _ _ _ _ _] -> w584
            tunnel: [_ _ _ _ _ w633 _ _ _ _ _ _ _] -> w583
            tunnel: [_ _ _ _ _ _ w637 _ _ _ _ _ _] -> w582
            tunnel: [_ _ _ _ _ _ _ w641 _ _ _ _ _] -> w581
            tunnel: [_ _ _ _ _ _ _ _ w645 _ _ _ _] -> w580
            tunnel: [_ _ _ _ _ _ _ _ _ w649 _ _ _] -> w579
            tunnel: w578 -> [_ _ _ _ _ _ _ _ _ _ w655 _ _]
            tunnel: [_ _ _ _ _ _ _ _ _ _ w654 _ _] -> w577
            tunnel: [_ _ _ _ _ _ _ _ _ _ _ w658 _] -> w576
            tunnel: w575 -> [_ _ _ _ _ _ _ _ _ _ _ w659 _]
            tunnel: [_ _ _ _ _ _ _ _ _ _ _ _ w664] -> w574
            tunnel: w573 -> [_ _ _ _ _ _ _ _ _ _ _ _ w663]
            tunnel: w571 -> [w601 w609 w617 w622 w627 w632 w636 w640 w644 w648 w652 w657 w662]
            tunnel: [_ _ w615 _ _ _ _ _ _ _ _ _ _] -> w572
            frame #0 {
              n166 = call-poly <vilib>:"Read Key.vi"("section"=w602, "key"=w601, "refnum"=w605) -> ("value"=w606:string)  [unwired: 5 in, 3 out]
              n167 = Search 1D Array(1D array=w607, element=w606) -> (index of element=w603:i32)  [unwired: 1 in]
              n168 = To Unsigned Word Integer(number=w603) -> (unsigned 16bit integer=w604:u16)
            }
            frame #1 {
              n169 = Concatenate Strings(w609, "x") -> (w608:string)
              n170 = call-poly <vilib>:"Read Key.vi"("section"=w613, "key"=w608, "refnum"=w614) -> ("value"=w612:dbl)  [unwired: 5 in, 3 out]
              n171 = To Single Precision Float(number=w612) -> (single precision float=w611:sgl)
            }
            frame #2 {
              n172 = Concatenate Strings(w617, "+") -> (w616:string)
              n173 = call-poly <vilib>:"Read Key.vi"("section"=w620, "key"=w616, "refnum"=w621) -> ("value"=w619:dbl)  [unwired: 5 in, 3 out]
              n174 = To Single Precision Float(number=w619) -> (single precision float=w615:sgl)
            }
            frame #3 {
              n175 = call-poly <vilib>:"Read Key.vi"("section"=w624, "key"=w622, "refnum"=w626) -> ("value"=w625:dbl)  [unwired: 5 in, 3 out]
              n176 = To Single Precision Float(number=w625) -> (single precision float=w623:sgl)
            }
            frame #4 {
              n177 = call-poly <vilib>:"Read Key.vi"("section"=w629, "key"=w627, "refnum"=w631) -> ("value"=w630:dbl)  [unwired: 5 in, 3 out]
              n178 = To Single Precision Float(number=w630) -> (single precision float=w628:sgl)
            }
            frame #5 {
              n179 = call-poly <vilib>:"Read Key.vi"("section"=w634, "key"=w632, "refnum"=w635) -> ("value"=w633:dbl)  [unwired: 5 in, 3 out]
            }
            frame #6 {
              n180 = call-poly <vilib>:"Read Key.vi"("section"=w638, "key"=w636, "refnum"=w639) -> ("value"=w637:dbl)  [unwired: 5 in, 3 out]
            }
            frame #7 {
              n181 = call-poly <vilib>:"Read Key.vi"("section"=w642, "key"=w640, "refnum"=w643) -> ("value"=w641:dbl)  [unwired: 5 in, 3 out]
            }
            frame #8 {
              n182 = call-poly <vilib>:"Read Key.vi"("section"=w646, "key"=w644, "refnum"=w647) -> ("value"=w645:dbl)  [unwired: 5 in, 3 out]
            }
            frame #9 {
              n183 = call-poly <vilib>:"Read Key.vi"("section"=w650, "key"=w648, "refnum"=w651) -> ("value"=w649:dbl)  [unwired: 5 in, 3 out]
            }
            frame #10 {
              n184 = call-poly <vilib>:"Read Key.vi"("section"=w655, "key"=w652, "refnum"=w656) -> ("value"=w653:dbl)  [unwired: 5 in, 3 out]
              n185 = To Single Precision Float(number=w653) -> (single precision float=w654:sgl)
            }
            frame #11 {
              n186 = call-poly <vilib>:"Read Key.vi"("section"=w659, "key"=w657, "refnum"=w661) -> ("value"=w660:dbl)  [unwired: 5 in, 3 out]
              n187 = To Single Precision Float(number=w660) -> (single precision float=w658:sgl)
            }
            frame #12 {
              n188 = call-poly <vilib>:"Read Key.vi"("section"=w663, "key"=w662, "refnum"=w666) -> ("value"=w665:dbl)  [unwired: 5 in, 3 out]
              n189 = To Single Precision Float(number=w665) -> (single precision float=w664:sgl)
            }
          }
          n190 = global read "全局F参数.vi" "2#拨钮下上Pr"() -> (w598:T2)
          n191 = Bundle By Name(cluster=w598, "选择"=w597, "系数x"=w586, "上限"=w585, "下限"=w584, "Ymax"=w583, "Ymin"=w582, "点数"=w581, "起点"=w580, "终点"=w579, "上参考"=w577, "下参考"=w576, "基准"=w574, "系数+"=w572) -> (w596:T2)
          n192 = global write "全局F参数.vi" "2#拨钮下上Pr"(w596) -> ()
        }
        frame #5 {
          n193 = stacked-sequence {
            tunnel: w696 -> [w703 _ _ _ _ _ _ _ _ _ _ _ _]
            tunnel: w695 -> [w701 w710 w717 w722 w727 w731 w735 w739 w743 w747 w752 w757 w762]
            tunnel: [w700 _ _ _ _ _ _ _ _ _ _ _ _] -> w693
            tunnel: w691 -> [w698 _ _ _ _ _ _ _ _ _ _ _ _]
            tunnel: w690 -> [_ w709 w716 _ _ _ _ _ _ _ _ _ _]
            tunnel: w689 -> [_ _ _ w720 _ _ _ _ _ _ _ _ _]
            tunnel: w688 -> [_ _ _ _ w725 _ _ _ _ _ _ _ _]
            tunnel: w687 -> [_ _ _ _ _ _ _ w738 _ _ _ _ _]
            tunnel: w686 -> [_ _ _ _ _ w730 _ _ _ _ _ _ _]
            tunnel: w685 -> [_ _ _ _ _ _ w734 _ _ _ _ _ _]
            tunnel: w684 -> [_ _ _ _ _ _ _ _ w742 _ _ _ _]
            tunnel: w683 -> [_ _ _ _ _ _ _ _ _ w746 _ _ _]
            tunnel: [_ w707 _ _ _ _ _ _ _ _ _ _ _] -> w682
            tunnel: [_ _ _ w719 _ _ _ _ _ _ _ _ _] -> w681
            tunnel: [_ _ _ _ w724 _ _ _ _ _ _ _ _] -> w680
            tunnel: [_ _ _ _ _ w729 _ _ _ _ _ _ _] -> w679
            tunnel: [_ _ _ _ _ _ w733 _ _ _ _ _ _] -> w678
            tunnel: [_ _ _ _ _ _ _ w737 _ _ _ _ _] -> w677
            tunnel: [_ _ _ _ _ _ _ _ w741 _ _ _ _] -> w676
            tunnel: [_ _ _ _ _ _ _ _ _ w745 _ _ _] -> w675
            tunnel: w674 -> [_ _ _ _ _ _ _ _ _ _ w751 _ _]
            tunnel: [_ _ _ _ _ _ _ _ _ _ w750 _ _] -> w673
            tunnel: [_ _ _ _ _ _ _ _ _ _ _ w754 _] -> w672
            tunnel: w671 -> [_ _ _ _ _ _ _ _ _ _ _ w755 _]
            tunnel: [_ _ _ _ _ _ _ _ _ _ _ _ w760] -> w670
            tunnel: w669 -> [_ _ _ _ _ _ _ _ _ _ _ _ w759]
            tunnel: w667 -> [w697 w705 w713 w718 w723 w728 w732 w736 w740 w744 w748 w753 w758]
            tunnel: [_ _ w711 _ _ _ _ _ _ _ _ _ _] -> w668
            frame #0 {
              n194 = call-poly <vilib>:"Read Key.vi"("section"=w698, "key"=w697, "refnum"=w701) -> ("value"=w702:string)  [unwired: 5 in, 3 out]
              n195 = Search 1D Array(1D array=w703, element=w702) -> (index of element=w699:i32)  [unwired: 1 in]
              n196 = To Unsigned Word Integer(number=w699) -> (unsigned 16bit integer=w700:u16)
            }
            frame #1 {
              n197 = Concatenate Strings(w705, "x") -> (w704:string)
              n198 = call-poly <vilib>:"Read Key.vi"("section"=w709, "key"=w704, "refnum"=w710) -> ("value"=w708:dbl)  [unwired: 5 in, 3 out]
              n199 = To Single Precision Float(number=w708) -> (single precision float=w707:sgl)
            }
            frame #2 {
              n200 = Concatenate Strings(w713, "+") -> (w712:string)
              n201 = call-poly <vilib>:"Read Key.vi"("section"=w716, "key"=w712, "refnum"=w717) -> ("value"=w715:dbl)  [unwired: 5 in, 3 out]
              n202 = To Single Precision Float(number=w715) -> (single precision float=w711:sgl)
            }
            frame #3 {
              n203 = call-poly <vilib>:"Read Key.vi"("section"=w720, "key"=w718, "refnum"=w722) -> ("value"=w721:dbl)  [unwired: 5 in, 3 out]
              n204 = To Single Precision Float(number=w721) -> (single precision float=w719:sgl)
            }
            frame #4 {
              n205 = call-poly <vilib>:"Read Key.vi"("section"=w725, "key"=w723, "refnum"=w727) -> ("value"=w726:dbl)  [unwired: 5 in, 3 out]
              n206 = To Single Precision Float(number=w726) -> (single precision float=w724:sgl)
            }
            frame #5 {
              n207 = call-poly <vilib>:"Read Key.vi"("section"=w730, "key"=w728, "refnum"=w731) -> ("value"=w729:dbl)  [unwired: 5 in, 3 out]
            }
            frame #6 {
              n208 = call-poly <vilib>:"Read Key.vi"("section"=w734, "key"=w732, "refnum"=w735) -> ("value"=w733:dbl)  [unwired: 5 in, 3 out]
            }
            frame #7 {
              n209 = call-poly <vilib>:"Read Key.vi"("section"=w738, "key"=w736, "refnum"=w739) -> ("value"=w737:dbl)  [unwired: 5 in, 3 out]
            }
            frame #8 {
              n210 = call-poly <vilib>:"Read Key.vi"("section"=w742, "key"=w740, "refnum"=w743) -> ("value"=w741:dbl)  [unwired: 5 in, 3 out]
            }
            frame #9 {
              n211 = call-poly <vilib>:"Read Key.vi"("section"=w746, "key"=w744, "refnum"=w747) -> ("value"=w745:dbl)  [unwired: 5 in, 3 out]
            }
            frame #10 {
              n212 = call-poly <vilib>:"Read Key.vi"("section"=w751, "key"=w748, "refnum"=w752) -> ("value"=w749:dbl)  [unwired: 5 in, 3 out]
              n213 = To Single Precision Float(number=w749) -> (single precision float=w750:sgl)
            }
            frame #11 {
              n214 = call-poly <vilib>:"Read Key.vi"("section"=w755, "key"=w753, "refnum"=w757) -> ("value"=w756:dbl)  [unwired: 5 in, 3 out]
              n215 = To Single Precision Float(number=w756) -> (single precision float=w754:sgl)
            }
            frame #12 {
              n216 = call-poly <vilib>:"Read Key.vi"("section"=w759, "key"=w758, "refnum"=w762) -> ("value"=w761:dbl)  [unwired: 5 in, 3 out]
              n217 = To Single Precision Float(number=w761) -> (single precision float=w760:sgl)
            }
          }
          n218 = global read "全局F参数.vi" "2#拨钮上下Pr"() -> (w694:T2)
          n219 = Bundle By Name(cluster=w694, "选择"=w693, "系数x"=w682, "上限"=w681, "下限"=w680, "Ymax"=w679, "Ymin"=w678, "点数"=w677, "起点"=w676, "终点"=w675, "上参考"=w673, "下参考"=w672, "基准"=w670, "系数+"=w668) -> (w692:T2)
          n220 = global write "全局F参数.vi" "2#拨钮上下Pr"(w692) -> ()
        }
        frame #6 {
          n221 = call <vilib>:"Close Config Data.vi"("refnum"=w763) -> ()  [unwired: 9 in, 2 out]
        }
      }
    }
    frame Error {
      n222 = call <vilib>:"Close Config Data.vi"("write file if changed (T)"=FALSE, "refnum"=w765) -> ()  [unwired: 8 in, 2 out]
    }
  }
